vi "Request Loopback.vi"(6 "timeout in ms (-1)":i32=-1, 8 "error in (no error)":errorcluster, 9 "Request Message Data":variant, 10 "Request Message":string, 11 "Mock Process in":refnum<class "Mock Process.lvclass">) -> (0 "error out":errorcluster, 1 "Response Message Data":variant, 2 "Response Message":string, 3 "Mock Process out":refnum<class "Mock Process.lvclass">, 4 "Timed out?":bool)   [LabVIEW 2020, in "Mock Process.lvclass"]
uses:
  Mock Process.lvclass
  Mock Process.lvclass/Mock Process.ctl
  Framework/Process/Process.lvclass
  C:/git/astemes-triarc-framework/source/Framework/Process/Process.lvclass
  C:/git/astemes-triarc-framework/source/Framework/Base/Base.lvclass
  C:/git/astemes-triarc-framework/source/Framework/Configuration File/Configuration File.lvclass
  C:/git/astemes-triarc-framework/source/Framework/Configuration/Configuration.lvclass
  C:/git/astemes-triarc-framework/source/Framework/Error Handler Interface/Error Handler Interface.lvclass
  C:/git/astemes-triarc-framework/source/Framework/Logging/Logging.lvclass
  C:/git/astemes-triarc-framework/source/Framework Test Suite/Mock Process/Mock Process.lvclass
  C:/git/astemes-triarc-framework/source/Framework/Async Handler/Async Handler.lvclass
  C:/git/astemes-triarc-framework/source/Framework/Helper Loop/Helper Loop.lvclass
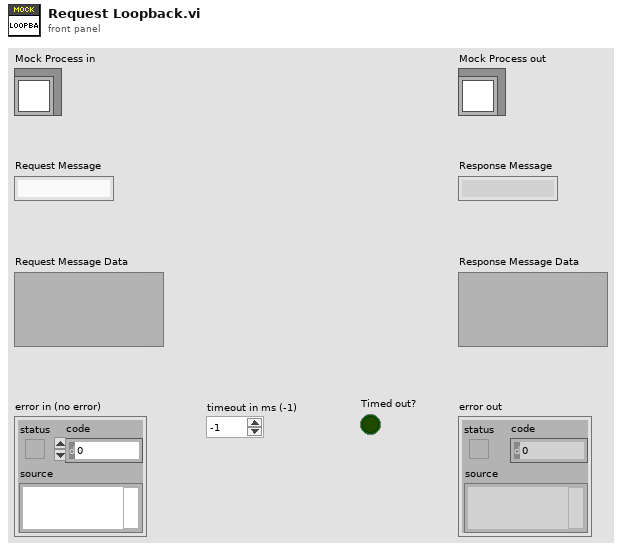
[diagram p1: front panel]
types:
  T1 = cluster{"Request Message":string, "Request Message Data":variant}
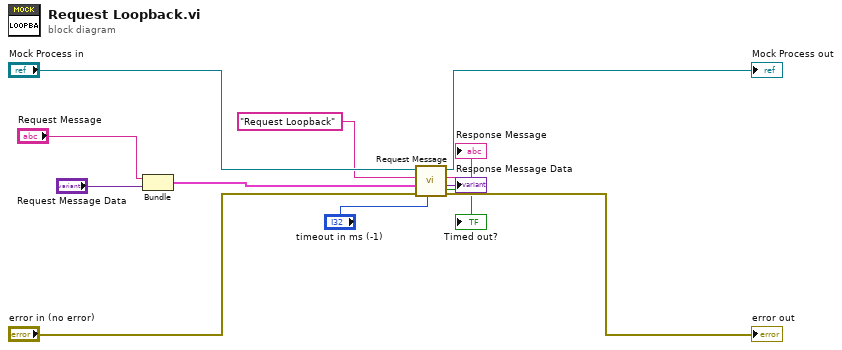
[diagram p0: block diagram]
diagram:
  n1 = Bundle("Request Message"="Request Message", "Request Message Data"="Request Message Data") -> (w3:T1)  [unwired: 1 in]
  n2 = call "Request Message.vi"("timeout in ms (-1)"="timeout in ms (-1)", "error in (no error)"="error in (no error)", "Request Message Data"=w3, "Request Message"="Request Loopback", "Process In"="Mock Process in") -> ("error out"=→"error out":errorcluster, "Response Message Data"=→"Response Message Data":variant, "Response Message"=→"Response Message":string, "Process Out"=→"Mock Process out":refnum<class "Mock Process.lvclass">, "Timed out?"=→"Timed out?":bool)  [unwired: 2 in]
